vi "Get Invalid DMA configurations.vi"(8 "error in (no error)":errorcluster, 10 "new bitfile dma configuration":T1[](array[typedef]) {"Data Type" format="%.0x"}, 11 "old bitfile dma configuration":T1[](array[typedef]) {"Data Type" format="%.0x"}) -> (0 "error out":errorcluster, 2 "still valid dma configurations":T1[](array[typedef]) {"Data Type" format="%.0x"}, 3 "invalid dma configurations":T1[](array[typedef]) {"Data Type" format="%.0x"})   [LabVIEW 2018]
uses:
  Addon Shared/Types/DMA Information.ctl
  Addon Shared/Types/Data Type.ctl
  Addon Shared/FPGA Addon Shared.lvlib
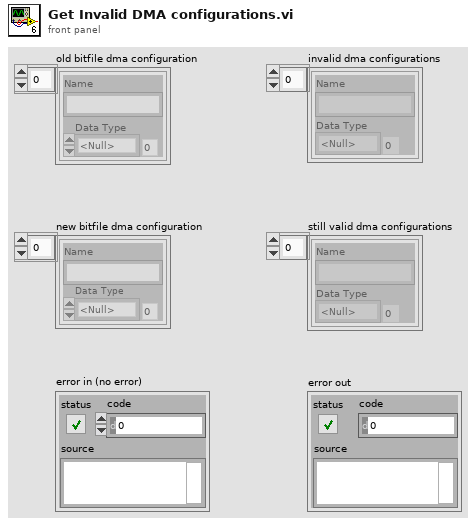
[diagram p1: front panel]
types:
  T1 = typedef "FPGA Addon Shared.lvlib/DMA Information.ctl" = cluster{"Name":string, "Data Type":T2}
  T2 = typedef "FPGA Addon Shared.lvlib/Data Type.ctl" = enum8{"<Null>", "I8", "I16", "I32", "I64", "U8", "U16", "U32", "U64", "SGL", "Boolean", "Analog PWM In Settings", "Analog PWM In", "Digital PWM In Settings", "Digital PWM In", "Digital PWM Out", "Sine Out", "FXP+/-24.5", "FXP+/-16.5", "FXP+/-32.8", "FXP+/-64.32", "FXP+/-16.7", "FXP+/-20.5", "FXP+/-27.5", "FXP+/-32.16", "FXP+16.3", "FXP+18.3", "Digital Static In", "Digital Static Out", "Digital Static In Settings", "Digital WSS Out", "Quad Encoder Settings", "Quad Encoder In", "Group"}
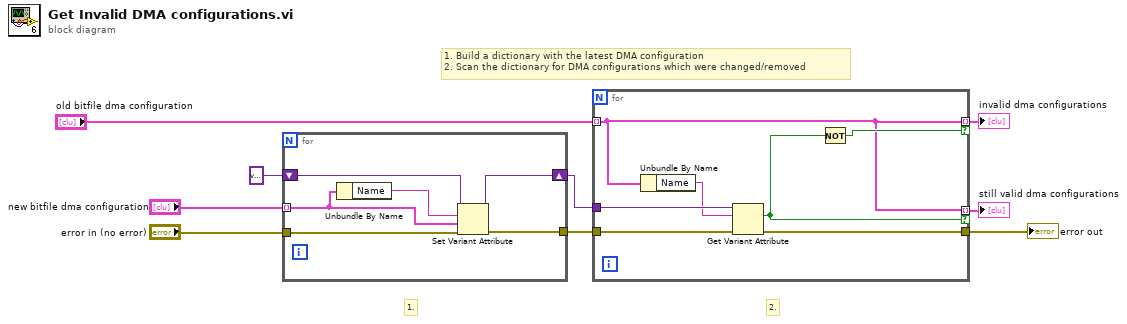
[diagram p0: block diagram]
diagram:
  # "1. Build a dictionary with the latest DMA configuration\n2. Scan the dictionary for DMA configurations which were changed/removed"
  # "2."
  # "1."
  n1 = for {
    tunnel: "new bitfile dma configuration" -> [w12] mode=indexing
    tunnel: "error in (no error)" -> [w14]
    tunnel: [w13] -> w7
    shift-right: [w10] -> w5
    shift-left: variant -> [w11]
    n2 = Unbundle By Name(w12) -> ("Name"=w15:string)
    n3 = Set Variant Attribute(Variant=w11, name=w15, value=w12, error in=w14) -> (Variant out=w10:variant, error out=w13:errorcluster)  [unwired: 1 out]
  }
  n4 = for {
    tunnel: [w19] -> w6
    tunnel: w7 -> [w22]
    tunnel: w5 -> [w21]
    tunnel: "old bitfile dma configuration" -> [w17] mode=indexing
    tunnel: [w17] -> w2 mode=indexing if=w18
    tunnel: [w17] -> w1 mode=indexing if=w16
    n5 = Unbundle By Name(w17) -> ("Name"=w20:string)
    n6 = Get Variant Attribute(Variant=w21, name=w20, error in=w22) -> (found=w16:bool, error out=w19:errorcluster)  [unwired: 1 in, 2 out]
    n7 = Not(x=w16) -> (.not. x?=w18:bool)
  }
  "error out" <- w6
  "invalid dma configurations" <- w2
  "still valid dma configurations" <- w1
